vi "Create Stacked Graph.vi"(1 "Y4":u16, 2 "Data":cluster{dbl[][]}[](array[cluster]), 3 "Y3":u16, 4 "Y2":u16, 5 "Y1":u16, 6 "X":u16) -> (0 "Graph":cluster{dbl[], dbl[]}[](array[cluster]))   [LabVIEW 2019]
panel:
  out "XY Graph":cluster{dbl[], dbl[]}[](graph)
  out "appended array":dbl[][](array[numeric])
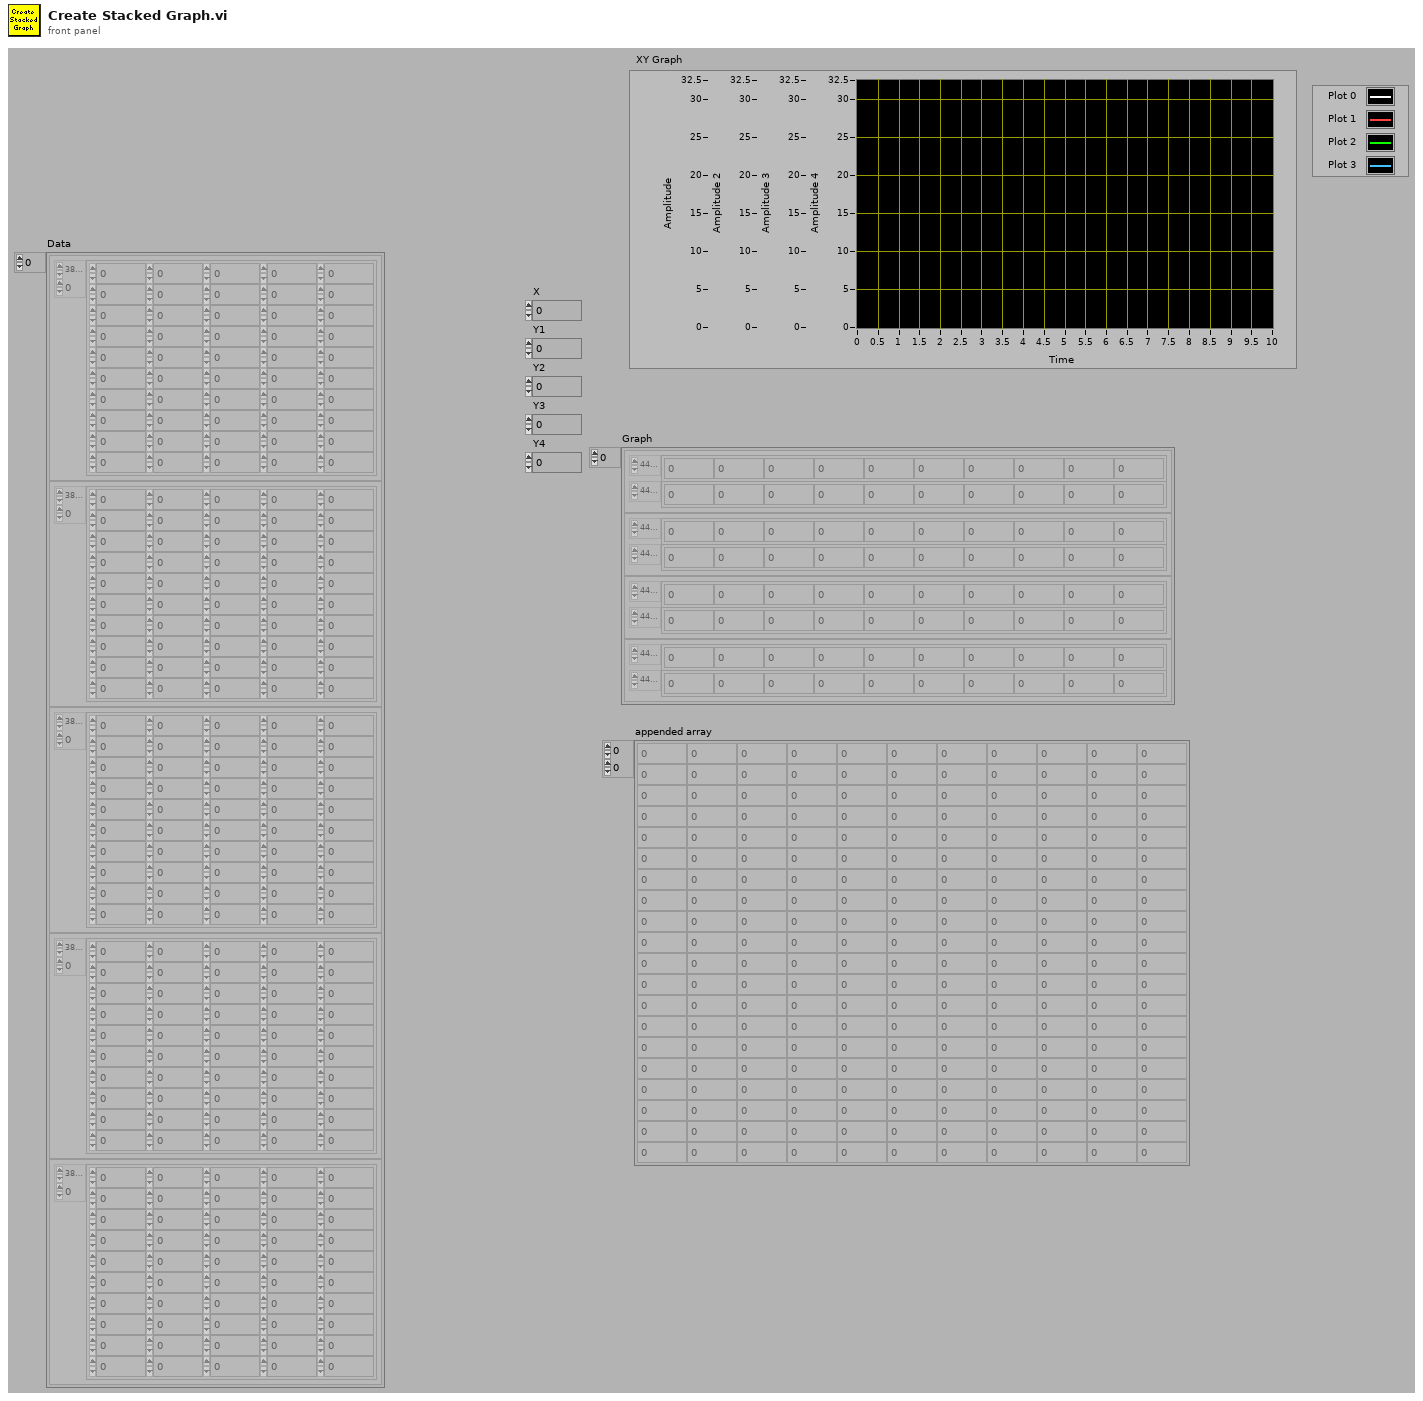
[diagram p1: front panel]
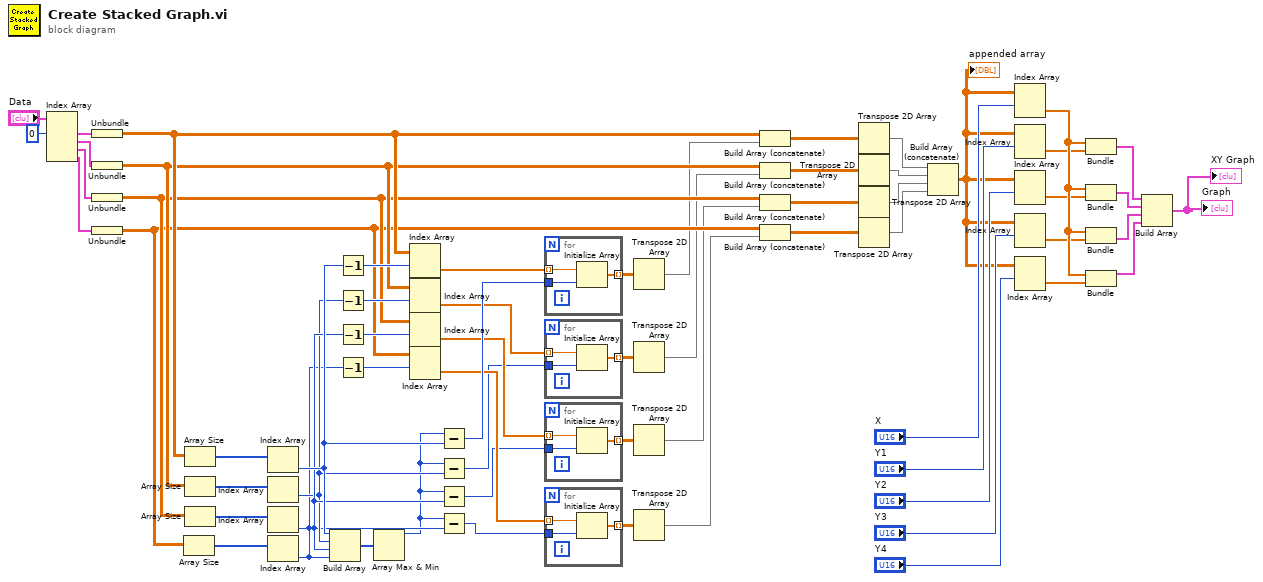
[diagram p0: block diagram]
diagram:
  n1 = Index Array(array="Data", index #1=0 ("index")) -> (element #1=w42:cluster{dbl[][]}, element #2=w43:cluster{dbl[][]}, element #3=w44:cluster{dbl[][]}, element #4=w45:cluster{dbl[][]})  [unwired: 3 in]
  n2 = Unbundle(w42) -> (w30:dbl[][])
  n3 = Unbundle(w43) -> (w29:dbl[][])
  n4 = Unbundle(w44) -> (w28:dbl[][])
  n5 = Unbundle(w45) -> (w27:dbl[][])
  n6 = Array Size(array=w27) -> (size(s)=w37:i32[])
  n7 = Array Size(array=w30) -> (size(s)=w35:i32[])
  n8 = Array Size(array=w29) -> (size(s)=w39:i32[])
  n9 = Array Size(array=w28) -> (size(s)=w38:i32[])
  n10 = Index Array(array=w35) -> (element=w5:i32)  [unwired: 1 in]
  n11 = Index Array(array=w39) -> (element=w3:i32)  [unwired: 1 in]
  n12 = Index Array(array=w38) -> (element=w4:i32)  [unwired: 1 in]
  n13 = Index Array(array=w37) -> (element=w2:i32)  [unwired: 1 in]
  n14 = Build Array(w5, w3, w4, w2) -> (w36:i32[])
  n15 = Decrement(x=w5) -> (x-1=w34:i32)
  n16 = Decrement(x=w3) -> (x-1=w33:i32)
  n17 = Decrement(x=w4) -> (x-1=w32:i32)
  n18 = Decrement(x=w2) -> (x-1=w31:i32)
  n19 = Array Max & Min(array=w36) -> (max value=w1:i32)  [unwired: 3 out]
  n20 = Index Array(array=w30, index (row)=w34) -> (element=w26:dbl[])  [unwired: 1 in]
  n21 = Index Array(array=w29, index (row)=w33) -> (element=w20:dbl[])  [unwired: 1 in]
  n22 = Index Array(array=w28, index (row)=w32) -> (element=w19:dbl[])  [unwired: 1 in]
  n23 = Index Array(array=w27, index (row)=w31) -> (element=w18:dbl[])  [unwired: 1 in]
  n24 = Subtract(x=w1, y=w5) -> (x-y=w21:i32)
  n25 = Subtract(x=w1, y=w3) -> (x-y=w17:i32)
  n26 = Subtract(x=w1, y=w4) -> (x-y=w16:i32)
  n27 = Subtract(x=w1, y=w2) -> (x-y=w15:i32)
  n28 = for {
    tunnel: w26 -> [w67] mode=indexing
    tunnel: w21 -> [w66]
    tunnel: [w65] -> w25 mode=indexing
    n29 = Initialize Array(w67, w66) -> (w65:dbl[])
  }
  n30 = for {
    tunnel: w20 -> [w70] mode=indexing
    tunnel: w17 -> [w69]
    tunnel: [w68] -> w24 mode=indexing
    n31 = Initialize Array(w70, w69) -> (w68:dbl[])
  }
  n32 = for {
    tunnel: w19 -> [w73] mode=indexing
    tunnel: w16 -> [w72]
    tunnel: [w71] -> w23 mode=indexing
    n33 = Initialize Array(w73, w72) -> (w71:dbl[])
  }
  n34 = for {
    tunnel: w18 -> [w76] mode=indexing
    tunnel: w15 -> [w75]
    tunnel: [w74] -> w22 mode=indexing
    n35 = Initialize Array(w76, w75) -> (w74:dbl[])
  }
  n36 = Transpose 2D Array(2D array=w25) -> (transposed array=w13:dbl[][])
  n37 = Transpose 2D Array(2D array=w24) -> (transposed array=w11:dbl[][])
  n38 = Transpose 2D Array(2D array=w23) -> (transposed array=w9:dbl[][])
  n39 = Transpose 2D Array(2D array=w22) -> (transposed array=w7:dbl[][])
  n40 = Build Array (concatenate)(w30, w13) -> (w14:dbl[][])
  n41 = Build Array (concatenate)(w29, w11) -> (w12:dbl[][])
  n42 = Build Array (concatenate)(w28, w9) -> (w10:dbl[][])
  n43 = Build Array (concatenate)(w27, w7) -> (w8:dbl[][])
  n44 = Transpose 2D Array(2D array=w14) -> (transposed array=w46:dbl[][])
  n45 = Transpose 2D Array(2D array=w12) -> (transposed array=w47:dbl[][])
  n46 = Transpose 2D Array(2D array=w10) -> (transposed array=w48:dbl[][])
  n47 = Transpose 2D Array(2D array=w8) -> (transposed array=w49:dbl[][])
  n48 = Build Array (concatenate)(w46, w47, w48, w49) -> (w50:dbl[][])
  "appended array" <- w50
  n49 = Index Array(array=w50, index (row)="X") -> (element=w55:dbl[])  [unwired: 1 in]
  n50 = Index Array(array=w50, index (row)="Y1") -> (element=w51:dbl[])  [unwired: 1 in]
  n51 = Index Array(array=w50, index (row)="Y2") -> (element=w52:dbl[])  [unwired: 1 in]
  n52 = Index Array(array=w50, index (row)="Y3") -> (element=w53:dbl[])  [unwired: 1 in]
  n53 = Index Array(array=w50, index (row)="Y4") -> (element=w54:dbl[])  [unwired: 1 in]
  n54 = Bundle(w55, w51) -> (w57:cluster{dbl[], dbl[]})  [unwired: 1 in]
  n55 = Bundle(w55, w52) -> (w56:cluster{dbl[], dbl[]})  [unwired: 1 in]
  n56 = Bundle(w55, w53) -> (w58:cluster{dbl[], dbl[]})  [unwired: 1 in]
  n57 = Bundle(w55, w54) -> (w59:cluster{dbl[], dbl[]})  [unwired: 1 in]
  n58 = Build Array(w57, w56, w58, w59) -> (→"Graph" →"XY Graph":cluster{dbl[], dbl[]}[])
